vi "Load Configuration From File.vi"(8 "error in (no error)":errorcluster, 9 "Instance Name":string, 10 "Configuration Path":path, 11 "System Actor in":refnum<class "System Actor.lvclass">) -> (0 "error out":errorcluster, 3 "System Actor out":refnum<class "System Actor.lvclass">)   [LabVIEW 2013, in "Robot Actors.lvlib" / "System Actor.lvlib" / "System Actor.lvclass"]
uses:
  System Actor.lvclass
  System Actor.lvclass/System Actor.ctl
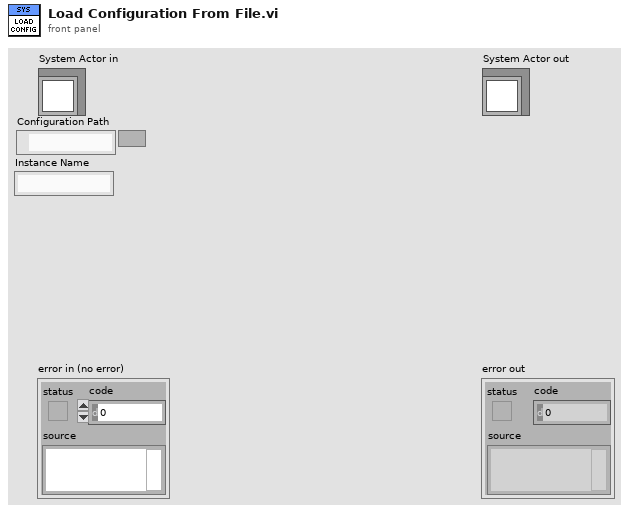
[diagram p1: front panel]
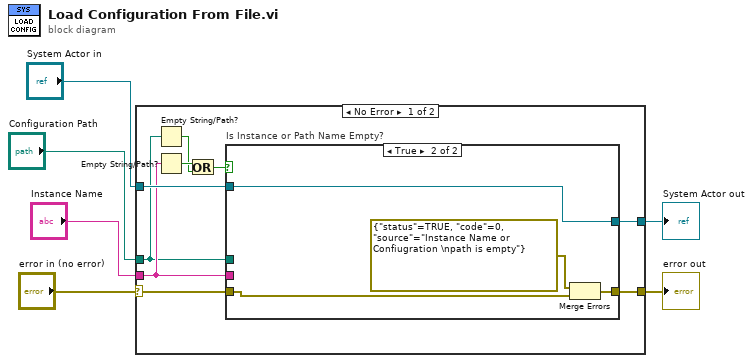
[diagram p0: block diagram]
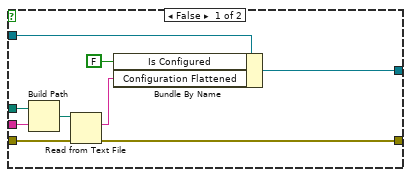
[diagram p2: hidden frame]
diagram:
  n1 = case shown="No Error" "error in (no error)" {
    selector: "error in (no error)" -> [w8 w30]
    tunnel: [w7 w30] -> w5
    tunnel: [w13 w29] -> w3
    tunnel: "System Actor in" -> [w15 w29]
    tunnel: "Configuration Path" -> [w12 _]
    tunnel: "Instance Name" -> [w14 _]
    frame No Error {
      n2 = Empty String/Path?(string/path=w12) -> (empty?=w10:bool)
      n3 = Empty String/Path?(string/path=w14) -> (empty?=w11:bool)
      n4 = Or(x=w11, y=w10) -> (x .or. y?=w9:bool)
      n5 = case "Is Instance or Path Name Empty?" shown="True" w9 {
        tunnel: w15 -> [w24 w25]
        tunnel: w12 -> [w23 _]
        tunnel: w14 -> [w19 _]
        tunnel: [w18 w25] -> w13
        tunnel: w8 -> [w17 w28]
        tunnel: [w16 w27] -> w7
        frame False {
          n6 = Build Path(base path=w23, name or relative path=w19) -> (appended path=w22:path)
          n7 = Read from Text File(file (use dialog)=w22, error in=w17) -> (text=w20:string, error out=w16:errorcluster)  [unwired: 2 in, 2 out]
          n8 = Bundle By Name(cluster=w24, "Is Configured"=FALSE, "Configuration Flattened"=w20) -> (w18:refnum<class "System Actor.lvclass">)
        }
        frame True {
          n9 = Merge Errors(errorcluster {"status"=TRUE, "code"=0, "source"="Instance Name or Confiugration \npath is empty"} ("error in"), w28) -> (w27:errorcluster)
        }
      }
    }
    frame Error {
    }
  }
  "error out" <- w5
  "System Actor out" <- w3
